vi "Extract Profile Array.vi"(8 "error in (no error)":errorcluster caption="エラー入力 (エラーなし)" {"code" format="%.0x"}, 9 "Profile Cnt":u32, 10 "Profile Data":u32[](array[numeric]), 11 "Profile Info":T1) -> (0 "error out":errorcluster caption="エラー出力" {"code" format="%.0x"}, 1 "Luminance Profile Array":u16[][](array[numeric]), 2 "Height Profile Array":dbl[][](array[numeric]), 3 "Header Array":u32[][](array[numeric]))   [LabVIEW 2020, in "KEYENCE LJ-X8000A.lvlib"]
doc: "Only height data of profiles without a header and footer will be extracted to output in two-dimensional array from profile data acquired with VI such as <B>Read Profiles</B> VI.\n\n<B>Note</B>:\nEmpty array will be output for corresponding output data if there is no profile data to extract."
uses:
  KEYENCE LJ-X8000A.lvlib
  Clusters/Profile Info.ctl
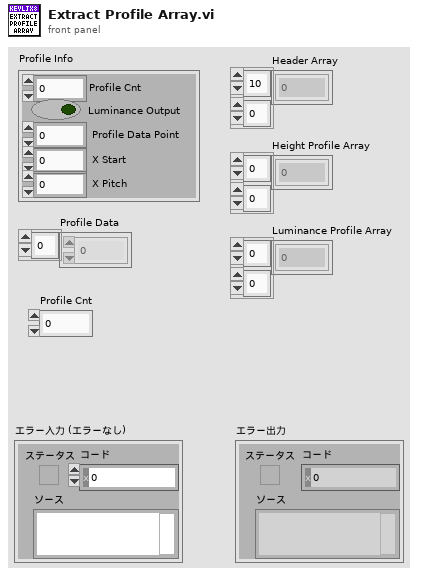
[diagram p1: front panel]
types:
  T1 = typedef "KEYENCE LJ-X8000A.lvlib/Profile Info.ctl" = cluster{"Profile Cnt":u8, "Luminance Output":bool, " Profile Data Point":u16, " X Start":i32, " X Pitch":i32}
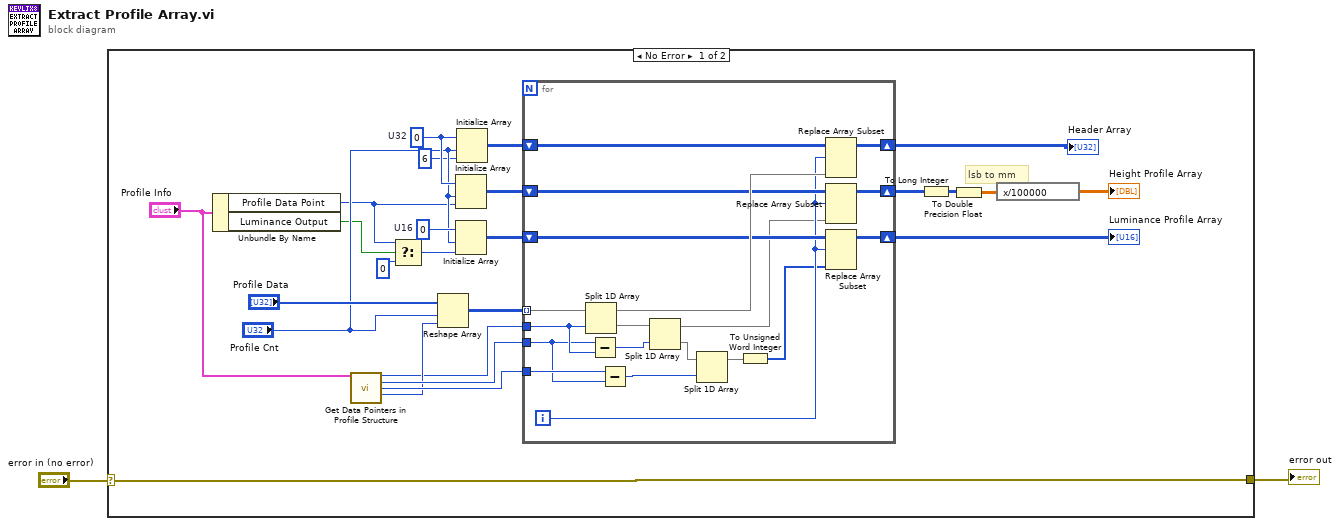
[diagram p0: block diagram]
diagram:
  n1 = case shown="No Error" "error in (no error)" {
    selector: "error in (no error)" -> [w20 w47]
    tunnel: [w20 w47] -> w1
    frame No Error {
      w16 = u16 0  # U16
      w17 = u32 0  # U32
      # "lsb to mm"
      n2 = Unbundle By Name("Profile Info") -> ("Profile Data Point"=w8:u16, "Luminance Output"=w9:bool)
      n3 = call "Get Data Pointers in Profile Structure.vi"("Profile Info"="Profile Info") -> ("Height Profile Pointer Index"=w22:u32, "Luminance Profile Pointer Index"=w24:u32, "Footer Pointer Index"=w25:u32, "Data Num of Raw Profile Structure"=w23:u32)  [unwired: 10 in, 1 out]
      n4 = Select(t=w8, s=w9, f=u16 0) -> (s? t:f=w6:u16)
      n5 = Reshape Array("Profile Data", "Profile Cnt", w23) -> (w21:u32[][])
      n6 = Initialize Array(w17, "Profile Cnt", w8) -> (w12:u32[][])
      n7 = Initialize Array(w16, "Profile Cnt", w6) -> (w11:u16[][])
      n8 = Initialize Array(w17, "Profile Cnt", 6 ("次元サイズ")) -> (w10:u32[][])
      n9 = for {
        tunnel: w21 -> [w46] mode=indexing
        tunnel: w22 -> [w43]
        tunnel: w24 -> [w41]
        tunnel: w25 -> [w42]
        shift-right: [w30] -> w5
        shift-left: w10 -> [w37]
        shift-right: [w29] -> w3
        shift-left: w12 -> [w35]
        shift-right: [w28] -> w4
        shift-left: w11 -> [w34]
        i -> [w33]
        n10 = Split 1D Array(array=w46, index=w43) -> (first subarray=w36:u32[], second subarray=w45:u32[])
        n11 = Subtract(x=w41, y=w43) -> (x-y=w44:u32)
        n12 = Subtract(x=w42, y=w41) -> (x-y=w40:u32)
        n13 = Split 1D Array(array=w45, index=w44) -> (first subarray=w32:u32[], second subarray=w39:u32[])
        n14 = Split 1D Array(array=w39, index=w40) -> (first subarray=w38:u32[])  [unwired: 1 out]
        n15 = To Unsigned Word Integer(number=w38) -> (unsigned 16bit integer=w31:u16[])
        n16 = Replace Array Subset(array=w37, new element=w36, index (row)=w33) -> (w30:u32[][])  [unwired: 1 in]
        n17 = Replace Array Subset(array=w35, new element=w32, index (row)=w33) -> (w29:u32[][])  [unwired: 1 in]
        n18 = Replace Array Subset(array=w34, new element=w31, index (row)=w33) -> (w28:u16[][])  [unwired: 1 in]
      }
      "Luminance Profile Array" <- w4
      "Header Array" <- w5
      n19 = To Long Integer(number=w3) -> (32bit integer=w18:i32[][])
      n20 = To Double Precision Float(number=w18) -> (double precision float=w26:dbl[][])
      n21 = expression code="x/100000"(w26) -> (→"Height Profile Array":dbl[][])
    }
    frame Error {
    }
  }
  "error out" <- w1
